vi "Init.vi"(8 "error in (no error)":errorcluster, 10 "Channel":i16, 11 "TrialBasedExperiment in":refnum<class "MultDimExperiment.lvclass">) -> (0 "error out":errorcluster, 3 "TrialBasedExperiment out":refnum<class "MultDimExperiment.lvclass">)   [LabVIEW 2012, in "MultDimExperiment.lvclass"]
uses:
  MultDimExperiment.lvclass
  Acquisition/AcquisitionCoreLibrary/AcquisitionCoreLibrary.lvlibp/labview-acquisition/Trial Based Experiment Statechart/PassiveExperiment/PassiveExperiment.lvclass
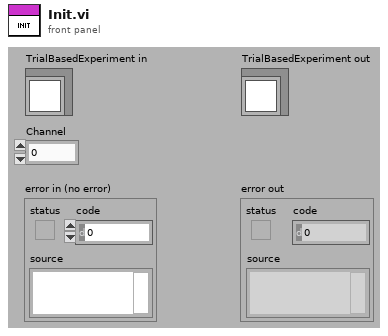
[diagram p1: front panel]
types:
  T1 = cluster{"Intertrial":dbl, "AcquireFixation":dbl, "HoldFixation":dbl, "DelayPeriod":dbl, "ResponsePeriod":dbl}
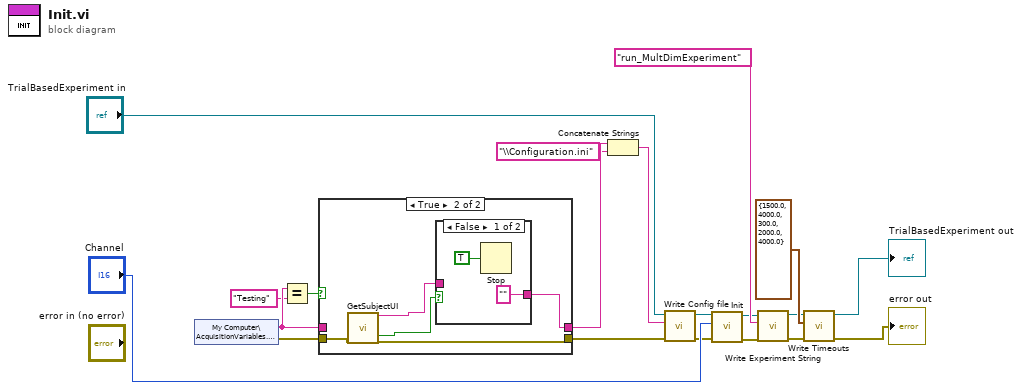
[diagram p0: block diagram]
diagram:
  n1 = shared-variable "My Computer\\AcquisitionVariables.lvlib\\Subject"() -> (w14:string, error out=w15:errorcluster)  [unwired: 1 in]
  n2 = Equal?(x=w14, y="Testing") -> (x = y?=w12:bool)
  n3 = case shown="True" w12 {
    tunnel: [w22 w27] -> w19
    tunnel: w14 -> [w22 _]
    tunnel: w15 -> [w21 w23]
    tunnel: [w21 w24] -> w16
    frame False {
    }
    frame True {
      n4 = call "GetSubjectUI.vi"("error in (no error)"=w23) -> ("subjectSelected"=w26:string, "OK"=w25:bool, "error out"=w24:errorcluster)  [unwired: 16 in]
      n5 = case shown="False" w25 {
        tunnel: w26 -> [_ w30]
        tunnel: ["" ("subjectSelected") w30] -> w27
        frame False {
          n6 = Stop(stop? (T)=TRUE) -> ()
        }
        frame True {
        }
      }
    }
  }
  n7 = Concatenate Strings(w19, "\\Configuration.ini") -> (w10:string)
  n8 = call-dynamic "Write Config file.vi"("error in (no error)"=w16, "Config file"=w10, "TrialBasedExperiment in"="TrialBasedExperiment in") -> ("error out"=w2:errorcluster, "TrialBasedExperiment out"=w6:refnum<class "MultDimExperiment.lvclass">)  [unwired: 7 in]
  n9 = call-parent "Init.vi"("error in (no error)"=w2, "Channel"="Channel", "TrialBasedExperiment in"=w6) -> ("error out"=w1:errorcluster, "TrialBasedExperiment out"=w5:refnum<class "MultDimExperiment.lvclass">)  [unwired: 7 in]
  n10 = call-dynamic "Write Experiment String.vi"("error in (no error)"=w1, "Experiment String"="run_MultDimExperiment" ("string"), "TrialBasedExperiment in"=w5) -> ("error out"=w9:errorcluster, "TrialBasedExperiment out"=w8:refnum<class "MultDimExperiment.lvclass">)  [unwired: 7 in]
  n11 = call-dynamic "Write Timeouts.vi"("error in (no error)"=w9, "Timeouts"=T1 {"Intertrial"=1500.0, "AcquireFixation"=4000.0, "HoldFixation"=300.0, "DelayPeriod"=2000.0, "ResponsePeriod"=4000.0}, "TrialBasedExperiment in"=w8) -> ("error out"=→"error out":errorcluster, "TrialBasedExperiment out"=→"TrialBasedExperiment out":refnum<class "MultDimExperiment.lvclass">)  [unwired: 7 in]
